vi "MES用户认证.vi"(8 "error in (no error)":errorcluster caption="错误输入（无错误）", 11 "MES配置":T1) -> (0 "error out":errorcluster caption="错误输出", 1 "RESULT":cluster{"Result":bool, "Message":string}, 3 "Data(OUT)":string="http://192.168.100.120:50000/manufacturing/IntegrationServlet?InterType=XML&message=<PRODUCTION_REQUEST><USER><SITE>A155</SITE><NAME>LTF</NAME><PWD>123456</PWD></USER></PRODUCTION_REQUEST>")   [LabVIEW 2011]
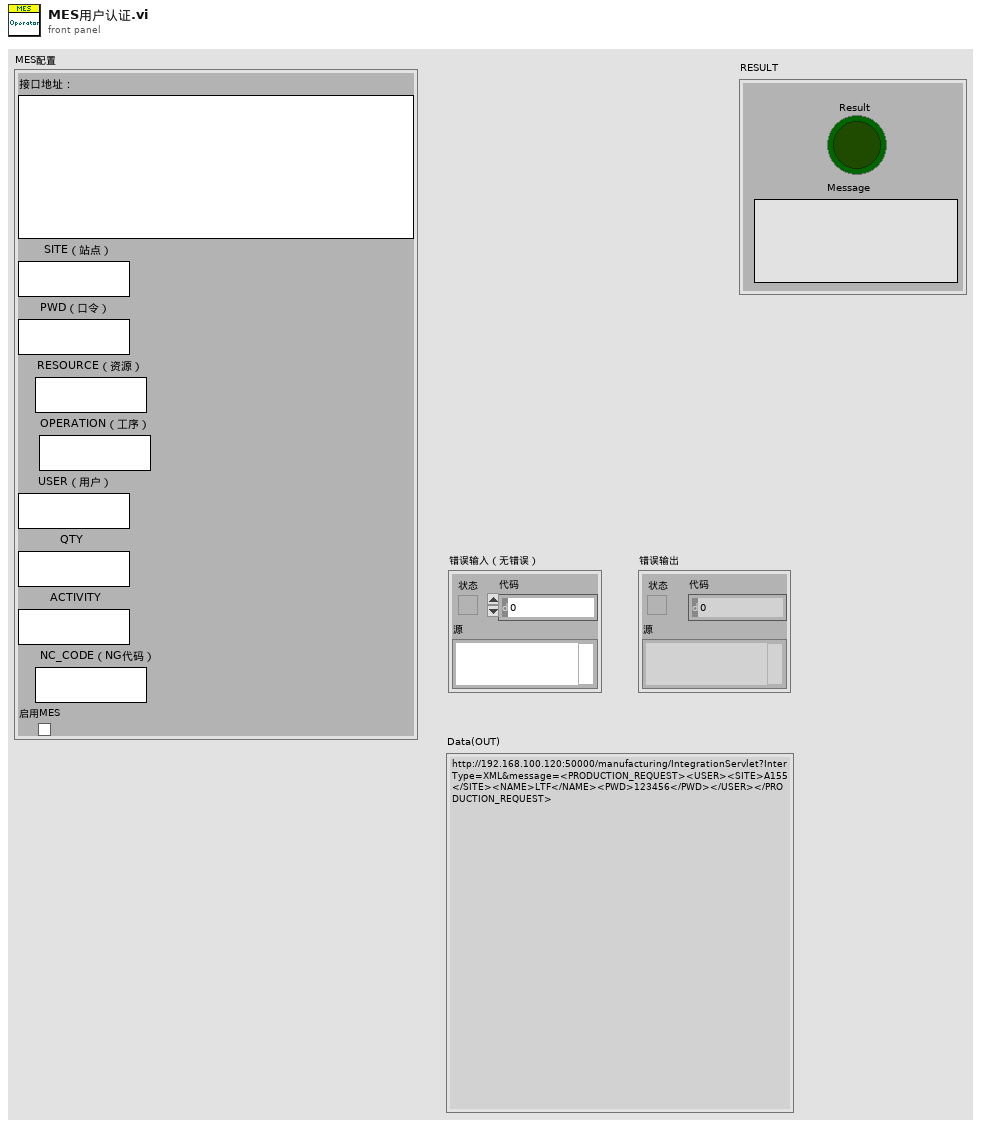
[diagram p1: front panel]
types:
  T1 = typedef "MES设置.ctl" = cluster{"接口地址：":string, "SITE（站点）   ":string, "PWD（口令）":string, "RESOURCE（资源）":string, "OPERATION（工序）":string, "USER（用户）":string, "QTY":string, "ACTIVITY":string, "NC_CODE（NG代码）":string, "启用MES":bool}
  T2 = enum16{"验证XML内容", "验证条码(Start)", "测试结果合格（PASS）", "测试结果不合格（ERROR）"}
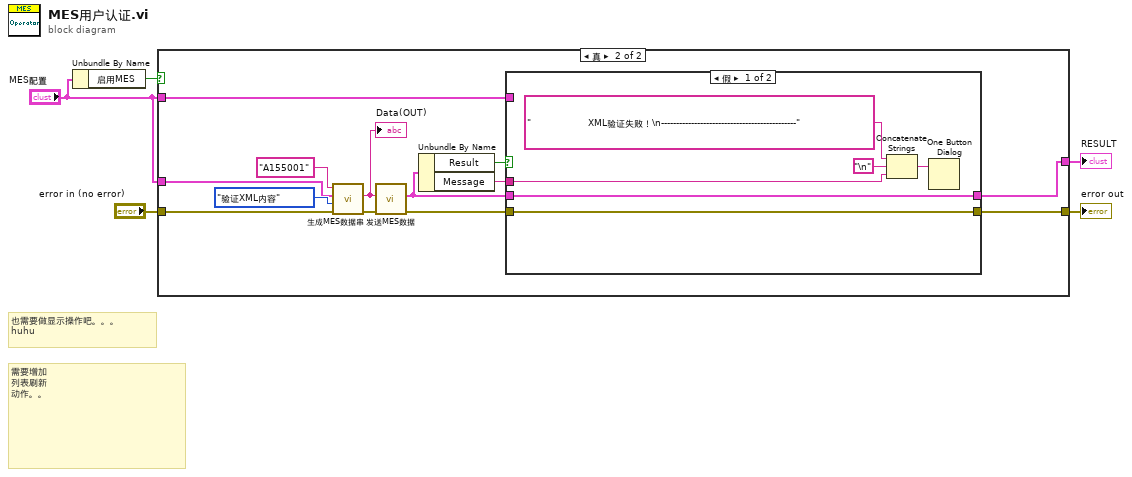
[diagram p0: block diagram]
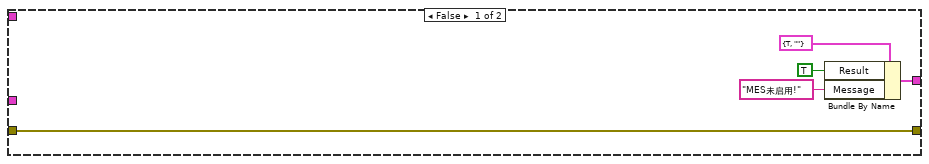
[diagram p2: hidden frame]
diagram:
  # "需要增加\n列表刷新\n动作。。"
  # "也需要做显示操作吧。。。\nhuhu"
  n1 = Unbundle By Name("MES配置") -> ("启用MES"=w2:bool)
  n2 = case shown="真" w2 {
    tunnel: "error in (no error)" -> [w6 w18]
    tunnel: [w6 w23] -> w4
    tunnel: [w7 w22] -> w3
    tunnel: "MES配置" -> [_ w13]
    tunnel: "MES配置" -> [_ w12]
    frame False {
      n3 = Bundle By Name(cluster=cluster{"Result":bool, "Message":string} {"Result"=TRUE, "Message"=""} ("RESULT"), "Result"=TRUE, "Message"="MES未启用!") -> (w7:cluster{"Result":bool, "Message":string})
    }
    frame True {
      n4 = call "生成MES数据串.vi"("error in (no error)"=w18, "操作状态"=T2."验证XML内容", "MES配置"=w13, "ID(SN)"="A155001") -> ("error out"=w19:errorcluster, "Data(OUT)"=w20:string)  [unwired: 6 in]
      "Data(OUT)" <- w20
      n5 = call "发送MES数据.vi"("error in (no error)"=w19, "Data(IN)"=w20) -> ("error out"=w17:errorcluster, "RESULT"=w14:cluster{"Result":bool, "Message":string})  [unwired: 6 in, 2 out]
      n6 = Unbundle By Name(w14) -> ("Result"=w16:bool, "Message"=w15:string)
      n7 = case shown="假" w16 {
        tunnel: [w24 w30] -> w23
        tunnel: [w25 w31] -> w22
        tunnel: w17 -> [w24 w30]
        tunnel: w15 -> [w26 _]
        tunnel: w14 -> [w25 w31]
        tunnel: w12 -> [_ _]
        frame False {
          n8 = Concatenate Strings("                   XML验证失败！\n---------------------------------------------", "\n", w26) -> (w28:string)
          n9 = One Button Dialog(message=w28) -> ()  [unwired: 1 in, 1 out]
        }
        frame True {
          # "通过\n验证"
        }
      }
    }
  }
  "error out" <- w4
  "RESULT" <- w3
